vi "fill_list.vi"(10 "Best 8":i32[][](array[numeric]), 11 "set max":cluster{"Channels":dbl[], "Intensity":dbl[]}) -> (3 "List Calibration":T1[](array[typedef]) {"Select Line" items=["Ka1", "Ka2", "Kb1", "La1", "La2", "Lb1", "Lb2", "Lg1"]; "Select Element" items=["Li", "Be", "B", "C", "N", "O", "F", "Ne", "Na", "Mg", "Al", "Si", "P", "S", "Cl", "Ar", "K", "Ca", "Sc", "Ti", "V", "Cr", "Mn", "Fe", "Co", "Ni", "Cu", "Zn", "Ga", "Ge", "As", "Se", "Br", "Kr", "Rb", "Sr", "Y", "Zr", "Nb", "Mo", "Tc", "Ru", "Rh", "Pd", "Ag", "Cd", "In", "Sn", "Sb", "Te", "I", "Xe", "Cs", "Ba", "La", "Ce", "Pr", "Nd", "Pm", "Sm", "Eu", "Gd", "Tb", "Dy", "Ho", "Er", "Tm", "Yb", "Lu", "Hf", "Ta", "W", "Re", "Os", "Ir", "Pt", "Au", "Hg", "Tl", "Pb", "Bi", "Po", "At", "Rn", "Fr", "Ra", "Ac", "Th", "Pa", "U", "Np", "Pu", "Am"]})   [LabVIEW 2023]
uses:
  control/calib.ctl
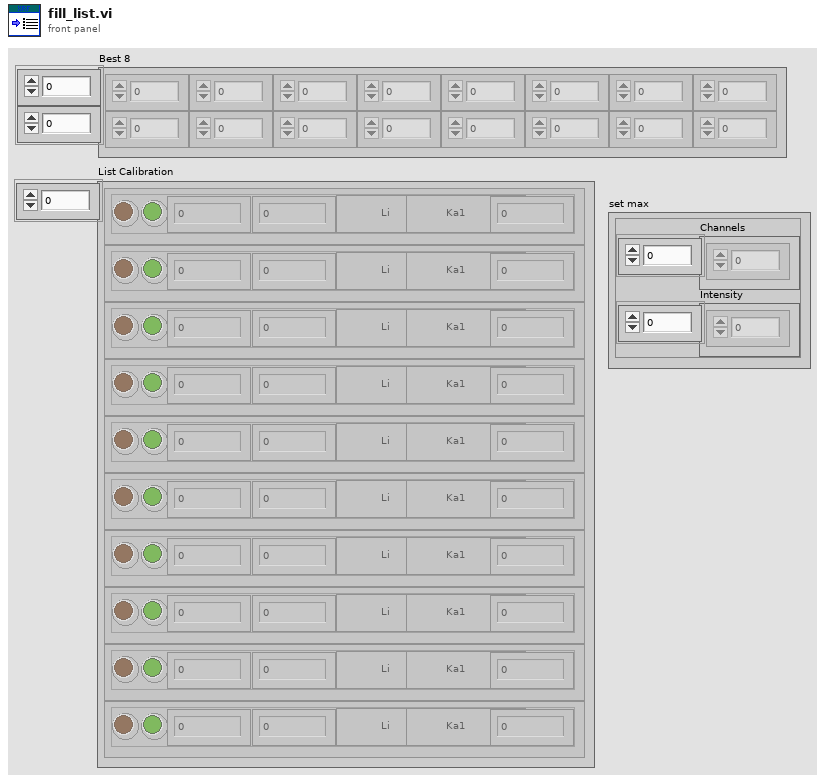
[diagram p1: front panel]
types:
  T1 = typedef "calib.ctl" = cluster{"select":bool, "Position":dbl, "Select Element":u16, "Select Line":u16, "Intensity":dbl, "Energy":dbl, "best":bool}
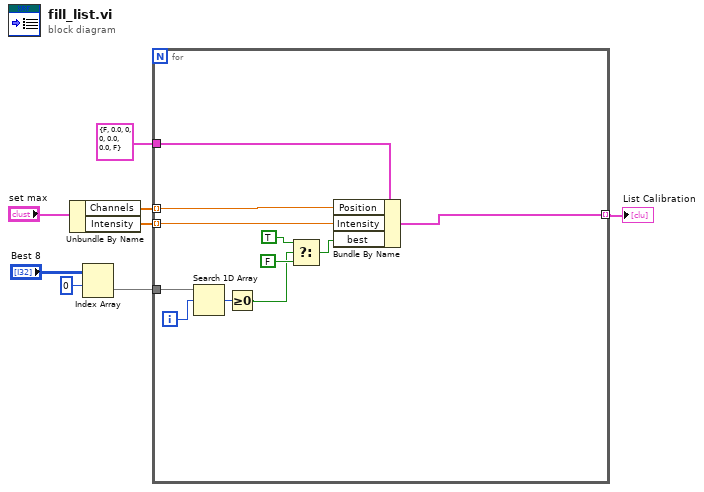
[diagram p0: block diagram]
diagram:
  n1 = Unbundle By Name("set max") -> ("Channels"=w7:dbl[], "Intensity"=w6:dbl[])
  n2 = Index Array(array="Best 8", index (row)=0) -> (element=w1:i32[])  [unwired: 1 in]
  n3 = for {
    tunnel: w7 -> [w17] mode=indexing
    tunnel: w6 -> [w18] mode=indexing
    tunnel: T1 {"select"=FALSE, "Position"=0.0, "Select Element"=0, "Select Line"=0, "Intensity"=0.0, "Energy"=0.0, "best"=FALSE} ("max peak") -> [w19]
    tunnel: [w16] -> w4 mode=indexing
    tunnel: w1 -> [w12]
    i -> [w11]
    n4 = Search 1D Array(1D array=w12, element=w11) -> (index of element=w10:i32)  [unwired: 1 in]
    n5 = Greater Or Equal To 0?(x=w10) -> (x >= 0?=w9:bool)
    n6 = Select(t=TRUE, s=w9, f=FALSE) -> (s? t:f=w13:bool)
    n7 = Bundle By Name(cluster=w19, "Position"=w17, "Intensity"=w18, "best"=w13) -> (w16:T1)
  }
  "List Calibration" <- w4
